vi "Parse GGA.vi"(8 "error in (no error)":errorcluster, 10 "Message":refnum<class "NMEA Message.lvclass">, 11 "nmea in":refnum<class "nmea.lvclass">) -> (0 "error out":errorcluster, 3 "nmea out":refnum<class "nmea.lvclass">)   [LabVIEW 2020, in "nmea.lvlib" / "nmea.lvclass"]
uses:
  nmea.lvclass
  message/NMEA Message.lvclass
  GGA Field.ctl
  nmea.lvclass/nmea.ctl
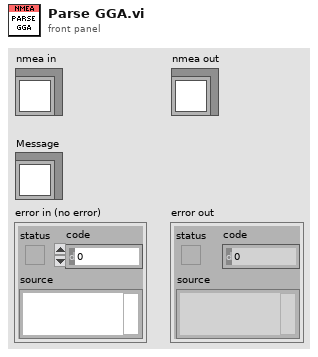
[diagram p1: front panel]
types:
  T1 = typedef "nmea.lvlib/nmea.lvclass/GGA Field.ctl" = enum16{"Time", "Latitude", "N/S", "Longitude", "E/W", "Quality", "Num Sats", "HDOP", "Altitude", "Geoid", "DGPS Age", "DGPS Station"}
  T2 = typedef "nmea.lvlib/nmea.lvclass/Ref Data.ctl" = cluster{"Latitude":dbl, "Longitude":dbl, "Time":T3, "Status":string, "Speed":dbl, "Course":dbl, "Mag Var":dbl, "Var Dir":string, "Mode":string, "Satellites":T4[], "Next Satellites":T4[], "Active PRNs":i32[], "Fix Type":T5, "DOP":T6, "Fix Mode":T7, "Altitude":dbl, "Geoid":dbl}
  T3 = typedef "LVDateTimeRec.ctl" = cluster{"fractional second":dbl, "second":i32, "minute":i32, "hour":i32, "day of month":i32, "month":i32, "year":i32, "day of week":i32, "day of year":i32, "DST":i32}
  T4 = typedef "nmea.lvlib/nmea.lvclass/Satellite.ctl" = cluster{"PRN":u8, "Channel":u8, "Elevation":u8, "Azimuth":u16, "SNR":u8, "Active":bool}
  T5 = typedef "nmea.lvlib/nmea.lvclass/Fix Type.ctl" = enum16{"N/A", "None", "2D", "3D"}
  T6 = typedef "nmea.lvlib/nmea.lvclass/DOP.ctl" = cluster{"P":dbl, "H":dbl, "V":dbl}
  T7 = typedef "nmea.lvlib/nmea.lvclass/Fix Mode.ctl" = enum16{"Manual", "Auto 2/3D"}
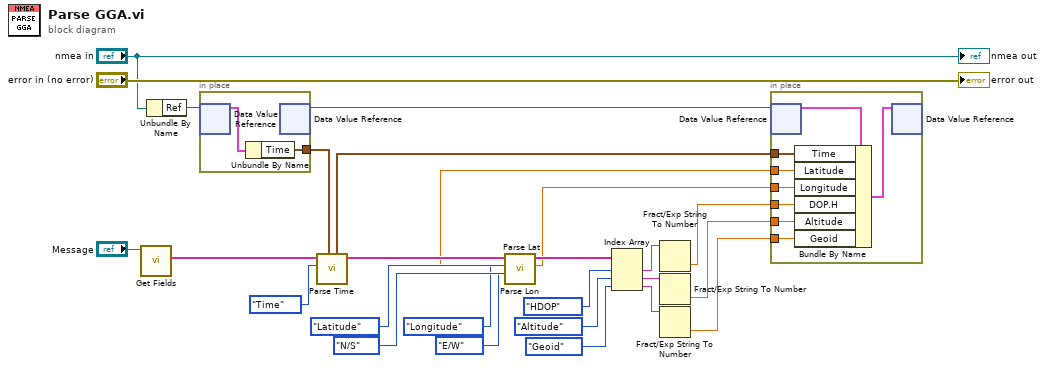
[diagram p0: block diagram]
diagram:
  n1 = call "Get Fields.vi"("NMEA Message in"="Message") -> ("Fields"=w25:string[])  [unwired: 8 in, 2 out]
  n2 = Unbundle By Name("nmea in") -> ("Ref"=w24:refnum<data-value>)
  n3 = in-place {
    in-place-border: [w28] -> w22
    n4 = in-place-dvr #1(w24) -> (w29:T2)  [unwired: 1 out]
    n5 = Unbundle By Name(w29) -> ("Time"=w28:T3)
    n6 = in-place-dvr #1() -> (w10:refnum<data-value>)  [unwired: 1 in, 1 out]
  }
  n7 = call "Parse Time.vi"("Time In"=w22, "Time Index"=GGA_Field."Time" ("GGA Field"), "Fields In"=w25) -> ("Fields"=w18:string[], "Time"=w9:T3)  [unwired: 7 in]
  n8 = call "Parse Lat.vi"("N/S Index"=GGA_Field."N/S" ("GGA Field"), "Latitude Index"=GGA_Field."Latitude" ("GGA Field"), "Fields In"=w18) -> ("Latitude"=w8:dbl, "Fields"=w17:string[])  [unwired: 7 in]
  n9 = call "Parse Lon.vi"("E/W Index"=GGA_Field."E/W" ("GGA Field"), "Longitude Index"=GGA_Field."Longitude" ("GGA Field"), "Fields In"=w17) -> ("Longitude"=w7:dbl, "Fields"=w14:string[])  [unwired: 7 in]
  n10 = Index Array(array=w14, index #1=GGA_Field."HDOP" ("GGA Field"), index #2=GGA_Field."Altitude" ("GGA Field"), index #3=GGA_Field."Geoid" ("GGA Field")) -> (element #1=w4:string, element #2=w6:string, element #3=w5:string)
  n11 = Fract/Exp String To Number(string=w4) -> (number=w3:dbl)  [unwired: 3 in, 1 out]
  n12 = Fract/Exp String To Number(string=w6) -> (number=w2:dbl)  [unwired: 3 in, 1 out]
  n13 = Fract/Exp String To Number(string=w5) -> (number=w1:dbl)  [unwired: 3 in, 1 out]
  n14 = in-place {
    in-place-border: w9 -> [w35]
    in-place-border: w8 -> [w34]
    in-place-border: w7 -> [w33]
    in-place-border: w3 -> [w32]
    in-place-border: w2 -> [w31]
    in-place-border: w1 -> [w30]
    n15 = in-place-dvr #2(w10) -> (w37:T2)  [unwired: 1 out]
    n16 = Bundle By Name(cluster=w37, "Time"=w35, "Latitude"=w34, "Longitude"=w33, "DOP.H"=w32, "Altitude"=w31, "Geoid"=w30) -> (w36:T2)
    n17 = in-place-dvr #2(w36) -> ()  [unwired: 2 out]
  }
  "error out" <- "error in (no error)"
  "nmea out" <- "nmea in"
